vi "Global for diagnostic.vi"() -> ()   [LabVIEW 2015]
panel:
  out "output cluster 2":T1
  out "speed out":cluster{i16, i16, i16, i16, i16, i16} {"?" scale=-32767.0..32767.0; "?" scale=-32767.0..32767.0; "?" scale=-32767.0..32767.0; "?" scale=-32767.0..32767.0; "?" scale=-32767.0..32767.0; "?" scale=-32767.0..32767.0}
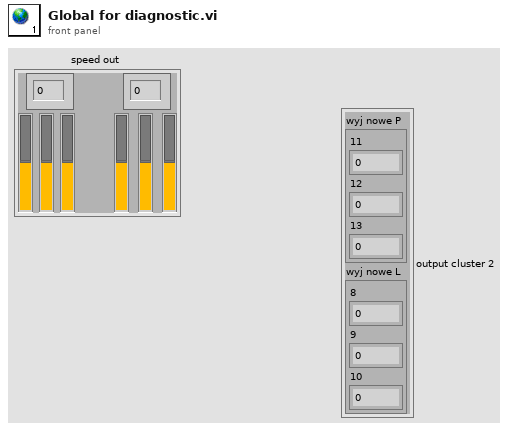
[diagram p1: front panel]
types:
  T1 = cluster{"wyj nowe P":cluster{"11":sgl, "12":sgl, "13":sgl}, "wyj nowe L ":cluster{"8":sgl, "9":sgl, "10":sgl}}
diagram:
